vi "transmit.vi"(8 "error in (no error)":errorcluster, 10 "RESP3 Value":variant, 11 "Redis Pipelining TCP Client in":refnum<class "Redis Pipelining TCP Client.lvclass">) -> (0 "error out":errorcluster, 3 "Redis Pipelining TCP Client out":refnum<class "Redis Pipelining TCP Client.lvclass">)   [LabVIEW 2019, in "Redis Client for LabVIEW.lvlib" / "Redis Pipelining TCP Client.lvclass"]
uses:
  Redis Pipelining TCP Client.lvclass
  Redis TCP Client/Redis TCP Client.lvclass
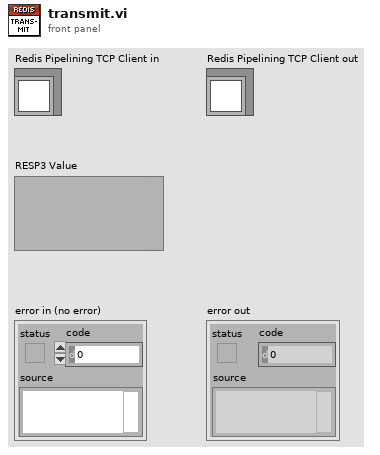
[diagram p1: front panel]
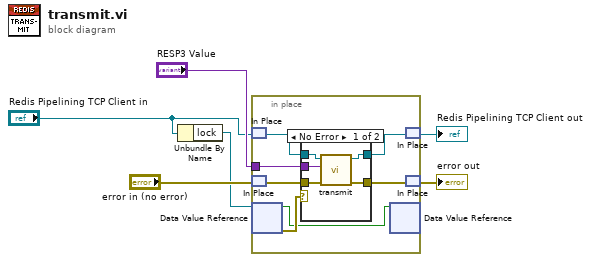
[diagram p0: block diagram]
diagram:
  n1 = Unbundle By Name("Redis Pipelining TCP Client in") -> ("lock"=w1:refnum<data-value>)
  n2 = in-place {
    in-place-border: "RESP3 Value" -> [w13]
    n3 = in-place-match #1("Redis Pipelining TCP Client in") -> (w11:refnum<class "Redis Pipelining TCP Client.lvclass">)
    n4 = in-place-match #2("error in (no error)") -> (w9:errorcluster)
    n5 = in-place-dvr #3(w1) -> (w7:bool, w8:errorcluster)
    n6 = case shown="No Error" w8 {
      selector: w8 -> [_ w20]
      tunnel: w13 -> [w17 _]
      tunnel: [w14 w19] -> w12
      tunnel: w11 -> [w18 w19]
      tunnel: w9 -> [w16 _]
      tunnel: [w15 w20] -> w10
      frame No Error {
        n7 = call-parent "transmit.vi"("error in (no error)"=w16, "RESP3 Value"=w17, "Redis TCP Client in"=w18) -> ("error out"=w15:errorcluster, "Redis TCP Client out"=w14:refnum<class "Redis Pipelining TCP Client.lvclass">)  [unwired: 7 in]
      }
      frame Error {
      }
    }
    n8 = in-place-dvr #3(w7) -> ()  [unwired: 2 out]
    n9 = in-place-match #1(w12) -> (→"Redis Pipelining TCP Client out":refnum<class "Redis Pipelining TCP Client.lvclass">)
    n10 = in-place-match #2(w10) -> (→"error out":errorcluster)
  }
